vi "minipampulse.vi"   [LabVIEW 2018]
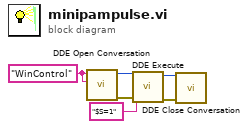
[diagram p0: block diagram]
diagram:
  w2 = "WinControl" ("service")
  n1 = call <vilib>:"DDE Open Conversation.vi"("topic"=w2, "service"=w2) -> ("error out"=w6:errorcluster, "conversation refnum"=w5:u32)  [unwired: 6 in]
  n2 = call <vilib>:"DDE Execute.vi"("error in (no error)"=w6, "command"="$S=1", "conversation refnum in"=w5) -> ("error out"=w4:errorcluster, "conversation refnum out"=w3:u32)  [unwired: 5 in]
  n3 = call <vilib>:"DDE Close Conversation.vi"("error in (no error)"=w4, "conversation refnum"=w3) -> ()  [unwired: 7 in, 1 out]
